vi "Read adjacency list item.vi"(5 "vertex":i32, 9 "DAG in":refnum<class "DAG.lvclass">) -> (3 "DAG out":refnum<class "DAG.lvclass">, 4 "edge list":i32[](array[numeric]))   [LabVIEW 2014, in "Raspberry Pi Compatible Compiler for LabVIEW.lvlib" / "DAG.lvclass"]
uses:
  DAG.lvclass
  DAG.lvclass/DAG.ctl
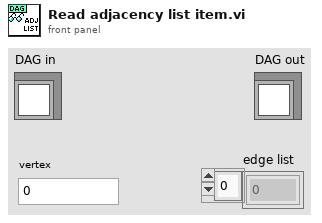
[diagram p1: front panel]
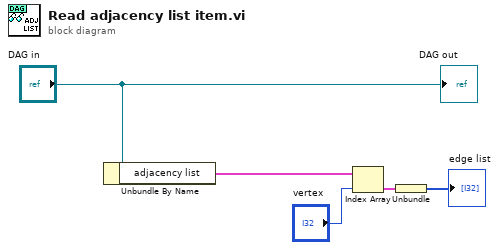
[diagram p0: block diagram]
diagram:
  n1 = Unbundle By Name("DAG in") -> ("adjacency list"=w4:cluster{"edge list":i32[]}[])
  n2 = Index Array(array=w4, index="vertex") -> (element=w2:cluster{"edge list":i32[]})
  n3 = Unbundle(w2) -> ("edge list"=→"edge list":i32[])
  "DAG out" <- "DAG in"
